vi "Test_EncloseSelection.vi"() -> ()   [LabVIEW 2025]
uses:
  8cebb4ce-4f0f-4319-9f7e-82e401bee674.vi
  ff6ee880-e87d-4ac2-b0b9-a7c0f406254d.vi
  57ba1f44-eecb-4af5-975d-0cda700306c1.vi
  Scripting Server.lvlib
panel:
  out "result":string
  out "error out":errorcluster
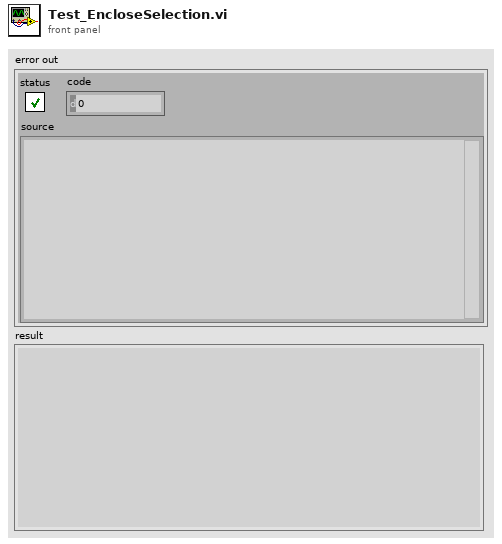
[diagram p1: front panel]
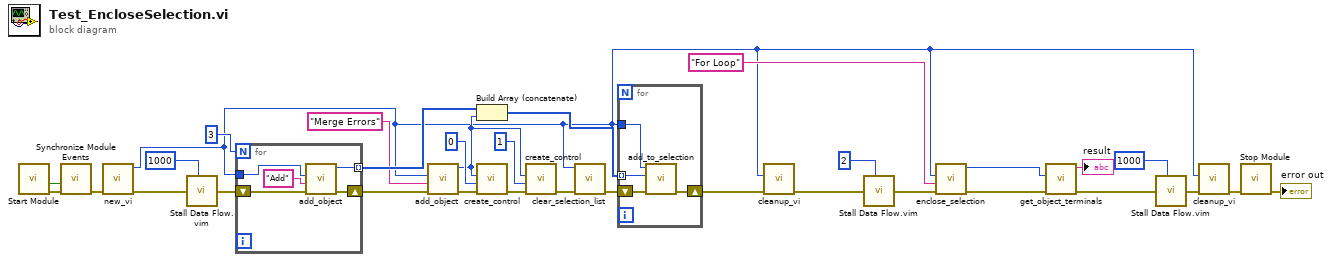
[diagram p0: block diagram]
diagram:
  n1 = call "Start Module.vi"() -> ("error out"=w31:errorcluster, "Wait for Event Sync?"=w32:bool)  [unwired: 7 in, 3 out]
  n2 = call "Synchronize Module Events.vi"("error in"=w31, "Wait for Event Sync?"=w32) -> ("error out"=w30:errorcluster)  [unwired: 9 in]
  n3 = call "new_vi.vi"("error in"=w30) -> ("error out"=w29:errorcluster, "vi_id"=w4:i32)  [unwired: 7 in, 2 out]
  n4 = call "Stall Data Flow.vim"("value in"=w29, "milliseconds to wait"=u32 1000) -> ("value out"=w28:errorcluster)  [unwired: 1 out]
  n5 = for {
    N: 3 -> [_]
    shift-right: [w36] -> w26
    shift-left: w28 -> [w37]
    tunnel: w4 -> [w33]
    tunnel: [w35] -> w25 mode=indexing
    n6 = call "add_object.vi"("error in"=w37, "object_name"="Add", "vi_reference"=w33) -> ("error out"=w36:errorcluster, "object_id"=w35:i32)  [unwired: 5 in, 2 out]
  }
  n7 = call "add_object.vi"("error in"=w26, "object_name"="Merge Errors", "vi_reference"=w4) -> ("error out"=w20:errorcluster, "object_id"=w12:i32)  [unwired: 5 in, 2 out]
  n8 = Build Array (concatenate)(w25, w12) -> (w11:i32[])
  n9 = call "create_control.vi"("error in"=w20, "terminal_index"=0, "object_id"=w12) -> ("error out"=w18:errorcluster)  [unwired: 6 in, 2 out]
  n10 = call "create_control.vi"("error in"=w18, "terminal_index"=1, "object_id"=w12) -> ("error out"=w16:errorcluster)  [unwired: 6 in, 2 out]
  n11 = call "clear_selection_list.vi"("error in"=w16, "vi_id"=w4) -> ("error out"=w14:errorcluster)  [unwired: 8 in, 1 out]
  n12 = for {
    tunnel: w4 -> [w39]
    tunnel: w11 -> [w38] mode=indexing
    shift-right: [w40] -> w13
    shift-left: w14 -> [w41]
    n13 = call "add_to_selection.vi"("error in"=w41, "object_id"=w38, "vi_id"=w39) -> ("error out"=w40:errorcluster)  [unwired: 7 in, 1 out]
  }
  n14 = call "cleanup_vi.vi"("error in"=w13, "vi_reference"=w4) -> ("error out"=w5:errorcluster)  [unwired: 7 in, 2 out]
  n15 = call "Stall Data Flow.vim"("value in"=w5, "milliseconds to wait"=u32 2) -> ("value out"=w8:errorcluster)  [unwired: 1 out]
  n16 = call "enclose_selection.vi"("error in"=w8, "structure_type"="For Loop", "vi_id"=w4) -> ("error out"=w10:errorcluster, "object_id"=w2:i32)  [unwired: 6 in, 1 out]
  n17 = call "get_object_terminals.vi"("error in"=w10, "object_id"=w2) -> ("error out"=w3:errorcluster, "result"=→"result":string)  [unwired: 7 in, 1 out]
  n18 = call "Stall Data Flow.vim"("value in"=w3, "milliseconds to wait"=u32 1000) -> ("value out"=w24:errorcluster)  [unwired: 1 out]
  n19 = call "cleanup_vi.vi"("error in"=w24, "vi_reference"=w4) -> ("error out"=w22:errorcluster)  [unwired: 7 in, 2 out]
  n20 = call "Stop Module.vi"("error in"=w22) -> ("error out"=→"error out":errorcluster)  [unwired: 10 in]
